vi "Execute-sequence.vi"(8 "error in (no error)":errorcluster, 9 "Activity log":refnum<user-event>, 10 "Abort":refnum<notifier>, 11 "Motor in":refnum<class "Motor.lvclass">) -> (0 "error out":errorcluster, 3 "Motor out":refnum<class "Motor.lvclass">)   [LabVIEW 2013, in "PowderDeposition.lvlib" / "Motor.lvclass"]
uses:
  Motor.lvclass
  Motor.lvclass/Motor.ctl
  Action/Action.lvclass
  Sequence/Action-sequence.lvclass
  Main/PD-Main.lvclass
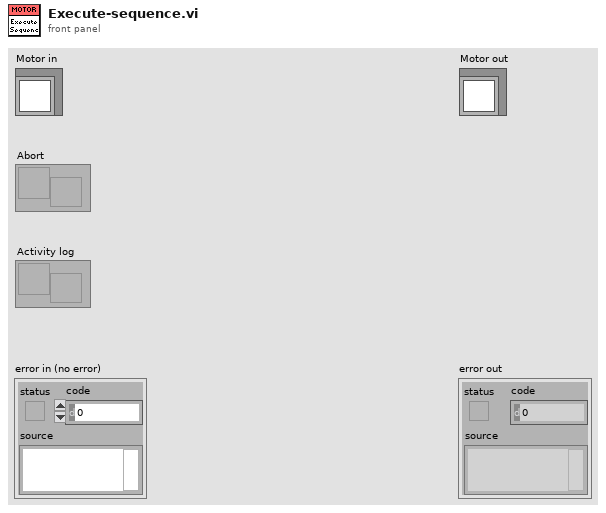
[diagram p1: front panel]
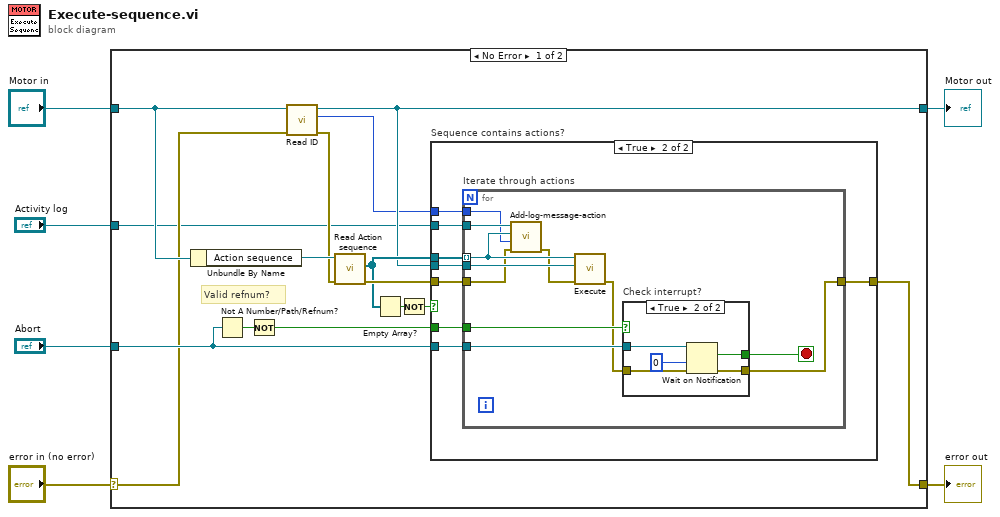
[diagram p0: block diagram]
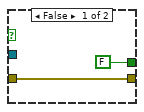
[diagram p3: hidden frame]
diagram:
  n1 = case shown="No Error" "error in (no error)" {
    selector: "error in (no error)" -> [w10 w50]
    tunnel: [w21 w50] -> w5
    tunnel: [w13 w49] -> w3
    tunnel: "Motor in" -> [w16 w49]
    tunnel: "Abort" -> [w11 _]
    tunnel: "Activity log" -> [w9 _]
    frame No Error {
      # "Valid refnum?"
      n2 = Unbundle By Name(w16) -> ("Action sequence"=w18:refnum<class "Action-sequence.lvclass">)
      n3 = Not A Number/Path/Refnum?(number/path/refnum=w11) -> (NaN/Path/Refnum?=w20:bool)
      n4 = Not(x=w20) -> (.not. x?=w19:bool)
      n5 = call-dynamic "Read ID.vi"("error in (no error)"=w10, "Motor in"=w16) -> ("error out"=w12:errorcluster, "ID"=w8:i32, "Motor out"=w13:refnum<class "Motor.lvclass">)  [unwired: 7 in]
      n6 = call "Read Action sequence.vi"("error in (no error)"=w12, "Sequence in"=w18) -> ("error out"=w17:errorcluster, "Action sequence"=w14:refnum<class "Action.lvclass">[])  [unwired: 7 in, 1 out]
      n7 = Empty Array?(array=w14) -> (empty?=w15:bool)
      n8 = Not(x=w15) -> (.not. x?=w7:bool)
      n9 = case "Sequence contains actions?" shown="True" w7 {
        tunnel: [w22 w30] -> w21
        tunnel: w11 -> [_ w29]
        tunnel: w19 -> [_ w28]
        tunnel: w14 -> [_ w27]
        tunnel: w17 -> [w22 w26]
        tunnel: w13 -> [_ w25]
        tunnel: w9 -> [_ w24]
        tunnel: w8 -> [_ w23]
        frame False {
        }
        frame True {
          n10 = for "Iterate through actions" {
            tunnel: w27 -> [w36] mode=indexing
            tunnel: w29 -> [w41]
            tunnel: w28 -> [w40]
            tunnel: w25 -> [w39]
            tunnel: w24 -> [w37]
            tunnel: w23 -> [w35]
            tunnel: w26 -> [w33]
            tunnel: [w32] -> w30
            stop <- w31 stop-if-true
            n11 = call "Add-log-message-action.vi"("error in (no error)"=w33, "Motor index"=w35, "Action"=w36, "Activity log"=w37) -> ("error out"=w34:errorcluster)  [unwired: 6 in, 1 out]
            n12 = call-dynamic "Execute.vi"("error in (no error)"=w34, "Motor in"=w39, "Action in"=w36) -> ("error out"=w38:errorcluster)  [unwired: 5 in, 3 out]
            n13 = case "Check interrupt?" shown="True" w40 {
              tunnel: w41 -> [_ w48]
              tunnel: w38 -> [w42 w47]
              tunnel: [w42 w46] -> w32
              tunnel: [FALSE w44] -> w31
              frame False {
              }
              frame True {
                n14 = Wait on Notification(notifier=w48, timeout in ms (-1)=0, error in (no error)=w47) -> (notification=w44:bool, error out=w46:errorcluster)  [unwired: 1 in, 2 out]
              }
            }
          }
        }
      }
    }
    frame Error {
    }
  }
  "error out" <- w5
  "Motor out" <- w3
